vi "B7_65.vi"(4 "error in":T13, 7 "Command":T14) -> (0 "error out":T13, 3 "Response":T11)   [LabVIEW 2018]
uses:
  MOKO_LabViewLibrary/MokoLowLevel/MokoLowLovelControl/MLLC_Command.ctl
  MOKO_LabViewLibrary/MokoLowLevel/MokoLowLovelControl/MLLC_Error.ctl
  MOKO_LabViewLibrary/MokoLowLevel/MokoLowLovelControl/MLLC_Mode.ctl
  MOKO_LabViewLibrary/MokoLowLevel/MokoLowLovelControl/MLLC_Response.ctl
  MOKO_LabViewLibrary/MokoLowLevel/MokoLowLovelControl/MLLC_DriverName.ctl
  MOKO_LabViewLibrary/MokoLowLevel/MokoLowLovelControl/MLLC_ErrorCode.ctl
  MOKO_LabViewLibrary/MokoLowLevel/MokoLowLovelControl/MLLC_Request.ctl
  MOKO_LabViewLibrary/MokoLowLevel/MokoLowLovelControl/MLLC_ResponseInit.ctl
  MOKO_LabViewLibrary/MokoLowLevel/MokoLowLovelControl/MLLC_ConnectCluster.ctl
  MOKO_LabViewLibrary/MokoLowLevel/MokoLowLovelControl/MLLC_InterfaceType.ctl
  MOKO_LabViewLibrary/MokoLowLevel/MokoLowLovelControl/MLLC_OpenedSession.ctl
  MOKO_LabViewLibrary/MokoLowLevel/MokoLowLovelControl/MLLC_InterfaceSettings.ctl
  MOKO_LabViewLibrary/MokoLowLevel/MokoLowLovelControl/MLLC_InterfaceKind.ctl
  MOKO_LabViewLibrary/MokoLowLevel/MokoLowLovelControl/MLLC_Rs232Settings.ctl
panel:
  in  "Settings":T7={"Data"={"Connect"={"InterfaceType"=enum."VISA", "OpenedSession"="COM1", "InterfaceSettings"={"Interface"=enum."RS232", "EOS 4 read"=enum."LF (\\n)", "EOS 4 write"=enum."LF (\\n)", "TMO, ms"=10000, "Sett"=variant(cluster{"Baud Rate":u32, "Data Bits":u16, "Parity":u16, "Stop Bits":u16, "Flow Control":u16, "Eho":bool} {"Baud Rate"=75, "Data Bits"=0, "Parity"=0, "Stop Bits"=0, "Flow Control"=0, "Eho"=FALSE})}}, "Delay, ms"=100, "Function"=enum."VDC", "DIGITS"=enum."1"}, "Saved Data"=variant}
  in  "ResponseInit":T8
  in  "Request":T9
  in  "Error Code":T6=5424
  in  "Driver Name":T10="B7_65"
  in  "Mode":T12=enum."Check"
  # "B7-65"
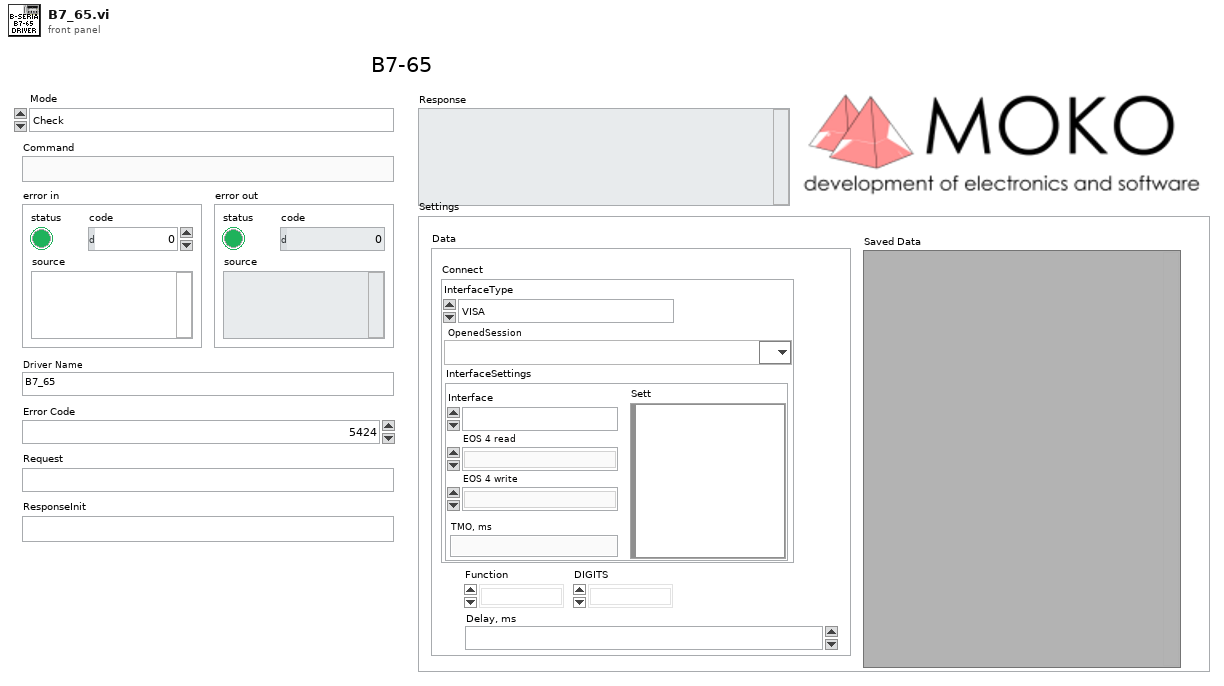
[diagram p1: front panel]
types:
  T1 = typedef "MLLC_ConnectCluster.ctl" = cluster{"InterfaceType":T2, "OpenedSession":T3, "InterfaceSettings":T4}
  T2 = typedef "MLLC_InterfaceType.ctl" = enum16{"VISA", "Prologix USB-GPIB"}
  T3 = typedef "MLLC_OpenedSession.ctl" = refnum<visa-resource-name>
  T4 = typedef "MLLC_InterfaceSettings.ctl" = cluster{"Interface":T5, "EOS 4 read":enum16{"Default (=EOS 4 write)", "CR (\\r)", "LF (\\n)", "None"}, "EOS 4 write":enum16{"CR+LF (\\r\\n)", "CR (\\r)", "LF (\\n)", "None"}, "TMO, ms":i32, "Sett":variant}
  T5 = typedef "MLLC_InterfaceKind.ctl" = enum16{"RS232", "GPIB", "USB", "Ethernet", "another"}
  T6 = typedef "MLLC_ErrorCode.ctl" = u32
  T7 = cluster{"Data":cluster{"Connect":T1, "Delay, ms":T6, "Function":enum16{"F", "T", "R4", "R", "IAC", "IDC", "VAC", "VDC"}, "DIGITS":enum16{"0", "1", "2"}}, "Saved Data":variant}
  T8 = typedef "MLLC_ResponseInit.ctl" = string
  T9 = typedef "MLLC_Request.ctl" = string
  T10 = typedef "MLLC_DriverName.ctl" = string
  T11 = typedef "MLLC_Response.ctl" = string
  T12 = typedef "MLLC_Mode.ctl" = enum16{"get", "set", "close", "Init", "Check"}
  T13 = typedef "MLLC_Error.ctl" = errorcluster
  T14 = typedef "MLLC_Command.ctl" = string
  T15 = cluster{"Connect":T1, "Delay, ms":T6, "Function":enum16{"F", "T", "R4", "R", "IAC", "IDC", "VAC", "VDC"}, "DIGITS":enum16{"0", "1", "2"}}
  T16 = enum16{"F", "T", "R4", "R", "IAC", "IDC", "VAC", "VDC"}
  T17 = typedef "MLLC_Rs232Settings.ctl" = cluster{"Baud Rate":u32, "Data Bits":u16, "Parity":u16, "Stop Bits":u16, "Flow Control":u16, "Eho":bool, "Address":dbl}
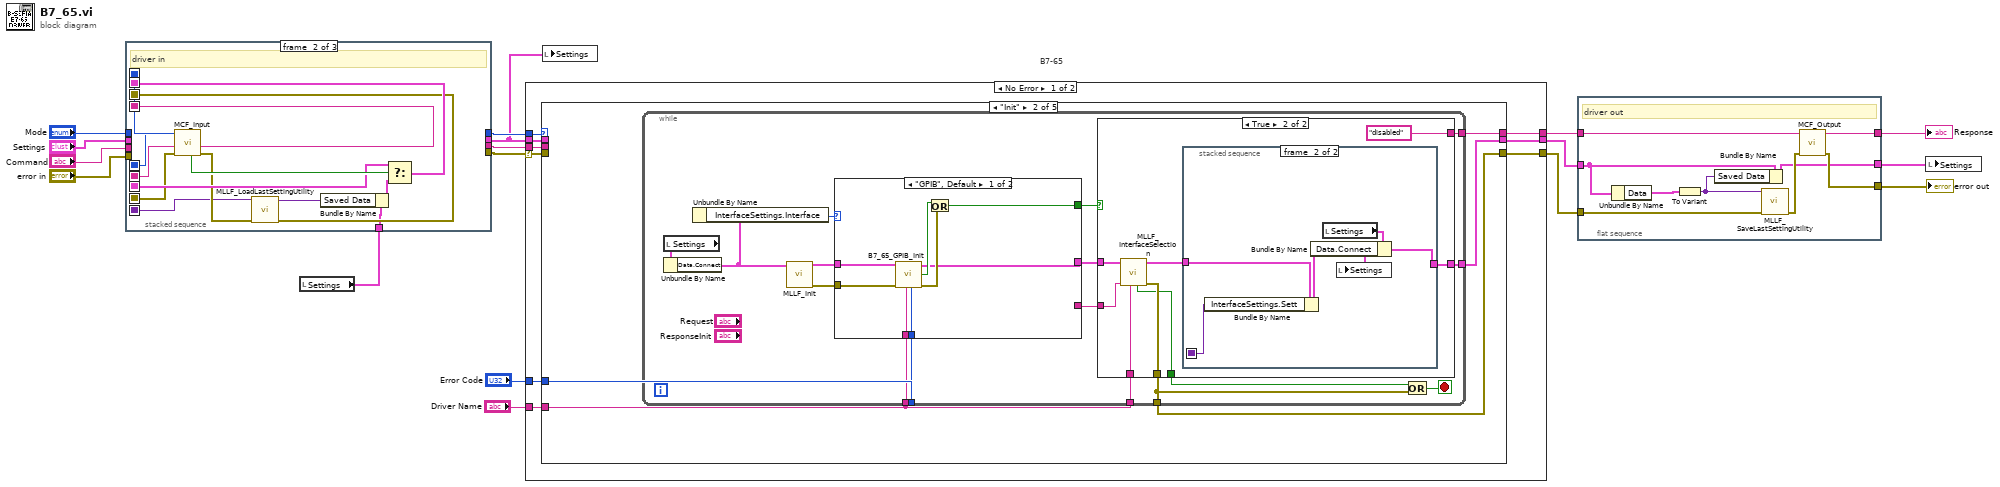
[diagram p0: block diagram]
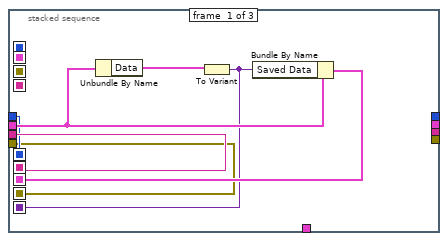
[diagram p2: hidden frame]
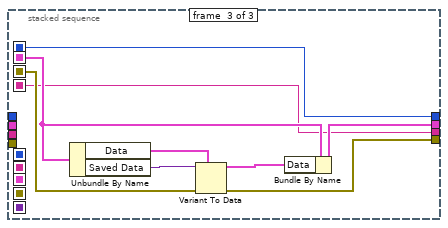
[diagram p3: hidden frame]
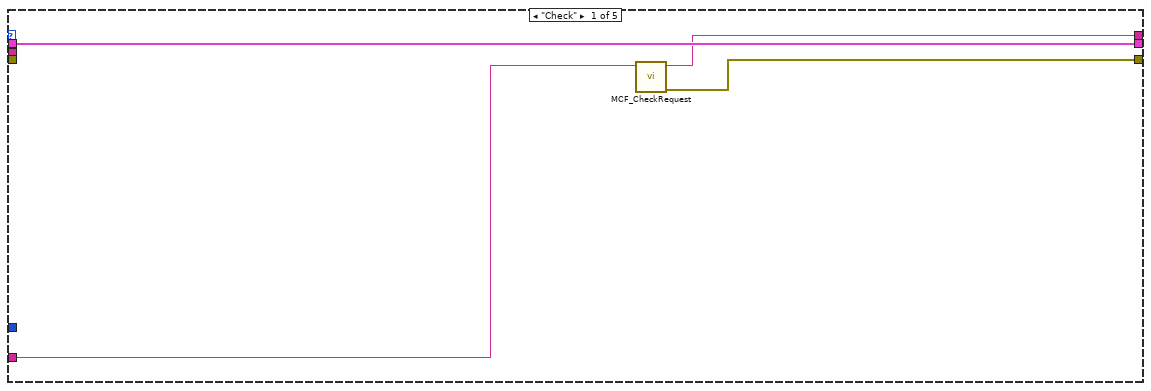
[diagram p4: hidden frame]
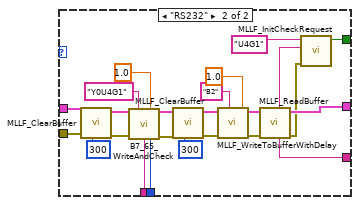
[diagram p5: hidden frame]
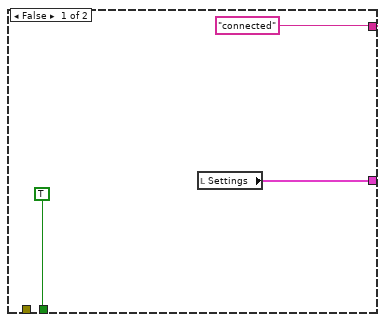
[diagram p6: hidden frame]
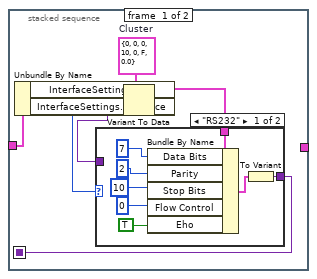
[diagram p7: hidden frame]
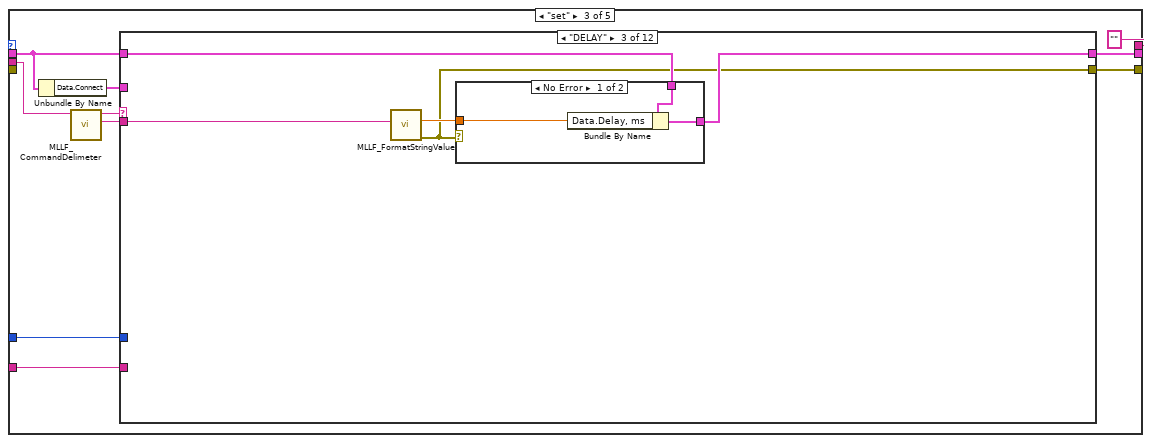
[diagram p9: hidden frame]
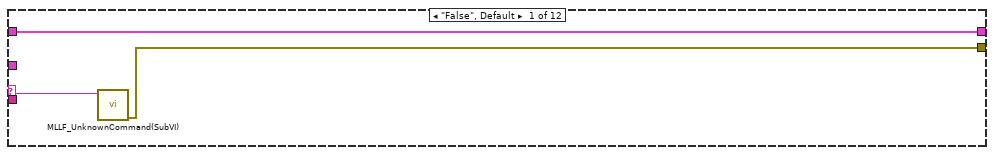
[diagram p10: hidden frame]
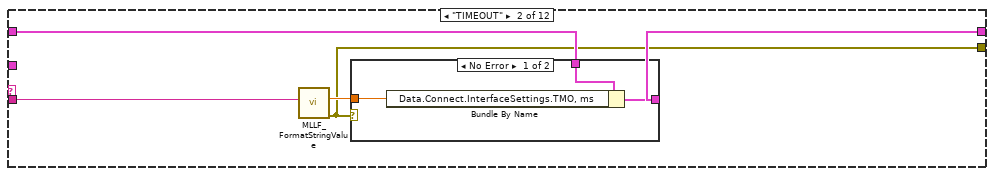
[diagram p11: hidden frame]
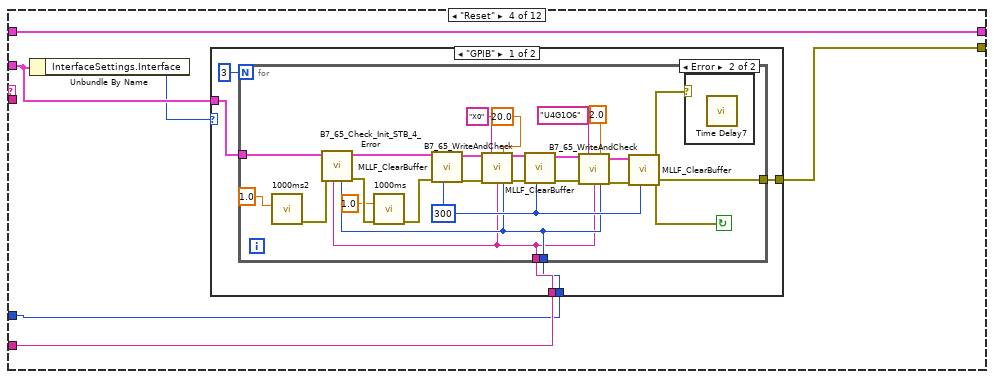
[diagram p14: hidden frame]
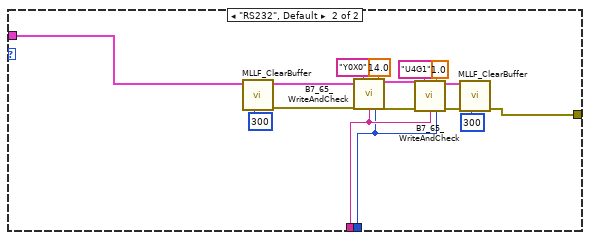
[diagram p16: hidden frame]
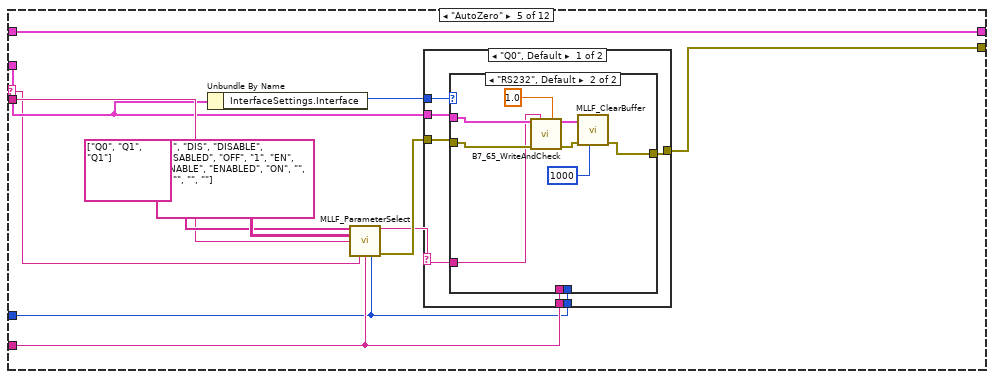
[diagram p17: hidden frame]
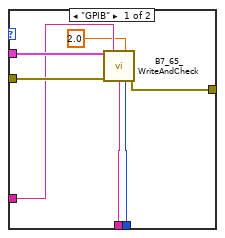
[diagram p18: hidden frame]
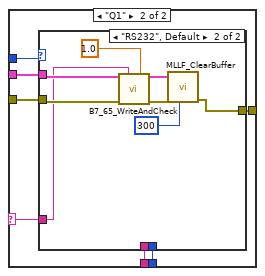
[diagram p19: hidden frame]
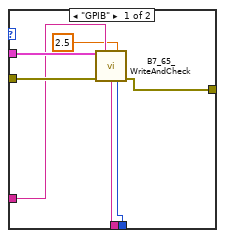
[diagram p20: hidden frame]
diagram:
  # "B7-65"
  n1 = local read "Settings"() -> (w11:T7)
  n2 = stacked-sequence {
    seq-local: [w20 _ _] -> [_ w36 _]
    seq-local: [w19 _ _] -> [_ w37 _]
    seq-local: [w22 _ _] -> [_ w32 _]
    seq-local: [w18 _ _] -> [_ w31 _]
    seq-local: [w21 _ _] -> [_ w27 _]
    seq-local: [_ w28 _] -> [_ _ w44]
    seq-local: [_ w38 _] -> [_ _ w41]
    seq-local: [_ w35 _] -> [_ _ w40]
    seq-local: [_ w34 _] -> [_ _ w45]
    tunnel: "Command" -> [w20 _ _]
    tunnel: "Mode" -> [w19 _ _]
    tunnel: "error in" -> [w18 _ _]
    tunnel: "Settings" -> [w23 _ _]
    tunnel: w11 -> [_ w26 _]
    tunnel: [_ _ w40] -> w8
    tunnel: [_ _ w43] -> w9
    tunnel: [_ _ w42] -> w7
    tunnel: [_ _ w41] -> w10
    frame #0 {
      n3 = Unbundle By Name(w23) -> ("Data"=w24:T15)
      n4 = To Variant(anything=w24) -> (Variant=w21:variant)
      n5 = Bundle By Name(cluster=w23, "Saved Data"=w21) -> (w22:T7)
    }
    frame #1 {
      # "driver in"
      n6 = call "MCF_Input.vi"("Error In"=w31, "Command in"=w36, "Mode in"=w37) -> ("Error Out"=w30:errorcluster, "Command out"=w35:string, "Mode out"=w38:T12, "Boolean"=w33:bool)  [unwired: 5 in]
      n7 = call "MLLF_LoadLastSettingUtility.vi"("Error In"=w30, "Save data in"=w27) -> ("Error Out"=w28:errorcluster, "Save data out"=w25:variant)  [unwired: 8 in]
      n8 = Bundle By Name(cluster=w26, "Saved Data"=w25) -> (w29:T7)
      n9 = Select(t=w32, s=w33, f=w29) -> (s? t:f=w34:T7)
    }
    frame #2 {
      n10 = Unbundle By Name(w45) -> ("Data"=w46:T15, "Saved Data"=w39:variant)
      n11 = Variant To Data(error in=w44, type=w46, Variant=w39) -> (data=w47:T15, error out=w42:errorcluster)
      n12 = Bundle By Name(cluster=w45, "Data"=w47) -> (w43:T7)
    }
  }
  n13 = case shown="No Error" w7 {
    selector: w7 -> [w52 w637]
    tunnel: [w54 w637] -> w4
    tunnel: w10 -> [w56 _]
    tunnel: [w55 _] -> w6
    tunnel: w8 -> [w53 _]
    tunnel: w9 -> [w49 w636]
    tunnel: "Error Code" -> [w51 _]
    tunnel: "Driver Name" -> [w50 _]
    tunnel: [w48 w636] -> w5
    frame No Error {
      n14 = case shown="\"Init\"" w56 {
        tunnel: [w59 w64 "" ("String") w417 "" ("String")] -> w55
        tunnel: [w58 w62 w144 w416 w634] -> w54
        tunnel: w53 -> [_ _ w153 w429 _]
        tunnel: w52 -> [_ _ _ _ _]
        tunnel: w51 -> [_ w65 w152 w426 _]
        tunnel: w50 -> [w57 w61 w149 w425 _]
        tunnel: w49 -> [w60 _ w151 w428 w633]
        tunnel: [w60 w63 w150 w427 w633] -> w48
        frame "Check" {
          n15 = call "MCF_CheckRequest.vi"("Driver Name"=w57) -> ("Error Out"=w58:errorcluster, "Output String"=w59:string)  [unwired: 9 in]
        }
        frame "Init" {
          n16 = while {
            tunnel: [w79] -> w62
            tunnel: w65 -> [w73]
            tunnel: w61 -> [w74]
            tunnel: [w71] -> w64
            tunnel: [w70] -> w63
            tunnel: w61 -> [w67]
            stop <- w78 stop-if-true
            n17 = local read "Settings"() -> (w81:T7)
            n18 = Unbundle By Name(w81) -> ("Data.Connect"=w68:T1)
            n19 = Unbundle By Name(w68) -> ("InterfaceSettings.Interface"=w72:T5)
            n20 = call "MLLF_Init.vi"("DriverConnect in"=w68) -> ("Error Out"=w75:errorcluster, "DriverConnect out"=w76:T1)  [unwired: 7 in]
            n21 = case shown="\"GPIB\", Default" w72 {
              tunnel: [w83 w112] -> w80
              tunnel: w76 -> [w88 w98]
              tunnel: w75 -> [w82 w97]
              tunnel: w74 -> [w87 w101]
              tunnel: w73 -> [w86 w100]
              tunnel: [w89 w93] -> w69
              tunnel: [_ w90] -> w66
              frame "GPIB", Default {
                n22 = call "B7_65_GPIB_Init.vi"("DriverConnect in"=w88, "error in"=w82, "Driver Name"=w87, "Error Code"=w86) -> ("DriverConnect out"=w83:T1, "Not Found response"=w84:bool, "error out"=w85:T13)  [unwired: 9 in]
                n23 = Or(x=w84, y=w85) -> (x .or. y?=w89:bool)
              }
              frame "RS232" {
                n24 = call "MLLF_ClearBuffer.vi"("Timeout(default = 300 ms)"=u32 300 ("Timeout"), "Error In"=w97, "DriverConnect in"=w98) -> ("Error Out"=w95:errorcluster, "DriverConnect out"=w96:T1)  [unwired: 5 in, 1 out]
                n25 = call "B7_65_WriteAndCheck.vi"("DriverConnect in"=w96, "Str2Write"="Y0U4G1" ("Request"), "Command Time (s)"=1.0, "error in"=w95, "Driver Name"=w101, "Error Code"=w100) -> ("DriverConnect out"=w104:T1, "error out"=w103:T13)  [unwired: 8 in]
                n26 = call "MLLF_ClearBuffer.vi"("Timeout(default = 300 ms)"=u32 300 ("Timeout"), "Error In"=w103, "DriverConnect in"=w104) -> ("Error Out"=w108:errorcluster, "DriverConnect out"=w109:T1)  [unwired: 5 in, 1 out]
                n27 = call "MLLF_WriteToBufferWithDelay.vi"("Delay Time ( 0,05 s)"=1.0 ("Command Time (s)"), "Command"="B2" ("Request"), "Error In"=w108, "DriverConnect in"=w109) -> ("Error Out"=w105:errorcluster, "DriverConnect out"=w106:T1)  [unwired: 6 in]
                n28 = call "MLLF_ReadBuffer.vi"("Error In"=w105, "DriverConnect in"=w106) -> ("Error Out"=w91:errorcluster, "DriverConnect out"=w112:T1, "String"=w90:string)  [unwired: 6 in]
                n29 = call "MLLF_InitCheckRequest.vi"("error in (no error)"=w91, "Answer"=w90, "Response Init"="U4G1" ("Response")) -> ("Design"=w93:bool)  [unwired: 5 in, 3 out]
              }
            }
            n30 = case shown="True" w69 {
              tunnel: w80 -> [_ w123]
              tunnel: [_ w121] -> w79
              tunnel: [TRUE w120] -> w77
              tunnel: [w113 w119] -> w70
              tunnel: ["connected" "disabled"] -> w71
              tunnel: w67 -> [_ w117]
              tunnel: w66 -> [_ w116]
              frame False {
                n31 = local read "Settings"() -> (w113:T7)
              }
              frame True {
                n32 = call "MLLF_InterfaceSelection.vi"("Driver Name"=w117, "Answer:"=w116, "DriverConnect in"=w123) -> ("error out"=w121:T13, "DriverConnect out"=w122:T1, "stop init?"=w120:bool)  [unwired: 4 in, 2 out]
                n33 = stacked-sequence {
                  seq-local: [w127 _] -> [_ w142]
                  tunnel: w122 -> [w124 w140]
                  tunnel: [_ w141] -> w119
                  frame #0 {
                    w129 = T17 {"Baud Rate"=0, "Data Bits"=0, "Parity"=0, "Stop Bits"=10, "Flow Control"=0, "Eho"=FALSE, "Address"=0.0}  # Cluster
                    n34 = Unbundle By Name(w124) -> ("InterfaceSettings.Sett"=w126:variant, "InterfaceSettings.Interface"=w125:T5)
                    n35 = Variant To Data(type=w129, Variant=w126) -> (data=w128:T17)  [unwired: 1 in, 1 out]
                    n36 = case shown="\"RS232\"" w125 {
                      tunnel: w128 -> [w136 _]
                      tunnel: [w137 w138] -> w127
                      tunnel: w126 -> [_ w138]
                      frame "RS232" {
                        n37 = Bundle By Name(cluster=w136, "Data Bits"=u16 7 ("Serial Settings:Data Bits"), "Parity"=u16 2 ("Flow Control"), "Stop Bits"=u16 10 ("Flow Control"), "Flow Control"=u16 0, "Eho"=TRUE) -> (w135:T17)
                        n38 = To Variant(anything=w135) -> (Variant=w137:variant)
                      }
                      frame "GPIB", Default {
                      }
                    }
                  }
                  frame #1 {
                    n39 = Bundle By Name(cluster=w140, "InterfaceSettings.Sett"=w142) -> (w139:T1)
                    n40 = local read "Settings"() -> (w143:T7)
                    n41 = Bundle By Name(cluster=w143, "Data.Connect"=w139) -> (w141:T7)
                    n42 = local write "Settings"(w141) -> ()
                  }
                }
              }
            }
            n43 = Or(x=w77, y=w79) -> (x .or. y?=w78:bool)
          }
        }
        frame "set" {
          n44 = Unbundle By Name(w151) -> ("Data.Connect"=w147:T1)
          n45 = call "MLLF_CommandDelimeter.vi"("command with param"=w153) -> ("param 1"=w145:string, "command"=w146:string)  [unwired: 6 in, 3 out]
          n46 = case shown="\"DELAY\"" w146 {
            selector: w146 -> [w155 _ _ _ w225 w281 _ w297 _ _ w378 w390]
            tunnel: w145 -> [_ w159 w168 _ w233 w291 _ w319 w333 _ w386 w404]
            tunnel: [w154 w157 w166 w180 w230 w288 _ w306 w334 _ w380 w393] -> w144
            tunnel: w152 -> [_ _ _ w177 w228 w286 _ w311 w339 _ w385 w400]
            tunnel: w151 -> [w156 w160 w169 w179 w236 w295 w296 w316 w351 w377 w389 w392]
            tunnel: [w156 w161 w170 w179 w236 w295 w296 w317 w351 w377 w389 w391] -> w150
            tunnel: w147 -> [_ _ _ w176 w226 w292 _ w298 w338 _ w383 w403]
            tunnel: w149 -> [_ _ _ w178 w229 w287 _ w312 w340 _ w384 w401]
            frame "False", Default {
              n47 = call "MLLF_UnknownCommand(SubVI).vi"("Unknown command"=w155) -> ("error out"=w154:errorcluster)  [unwired: 10 in]
            }
            frame "TIMEOUT" {
              n48 = call "MLLF_FormatStringValue.vi"("String Value"=w159) -> ("error out"=w157:T13, "number"=w158:dbl)  [unwired: 8 in, 1 out]
              n49 = case shown="No Error" w157 {
                tunnel: [w164 w165] -> w161
                tunnel: w160 -> [w163 w165]
                tunnel: w158 -> [w162 _]
                frame No Error {
                  n50 = Bundle By Name(cluster=w163, "Data.Connect.InterfaceSettings.TMO, ms"=w162) -> (w164:T7)
                }
                frame Error {
                }
              }
            }
            frame "DELAY" {
              n51 = call "MLLF_FormatStringValue.vi"("String Value"=w168) -> ("error out"=w166:T13, "number"=w167:dbl)  [unwired: 8 in, 1 out]
              n52 = case shown="No Error" w166 {
                tunnel: [w173 w174] -> w170
                tunnel: w169 -> [w172 w174]
                tunnel: w167 -> [w171 _]
                frame No Error {
                  n53 = Bundle By Name(cluster=w172, "Data.Delay, ms"=w171) -> (w173:T7)
                }
                frame Error {
                }
              }
            }
            frame "Reset" {
              n54 = Unbundle By Name(w176) -> ("InterfaceSettings.Interface"=w175:T5)
              n55 = case shown="\"GPIB\"" w175 {
                tunnel: w178 -> [w183 w218]
                tunnel: w177 -> [w182 w217]
                tunnel: [w185 w224] -> w180
                tunnel: w176 -> [w184 w209]
                frame "GPIB" {
                  n56 = for {
                    N: 3 -> [_]
                    tunnel: [w194] -> w185
                    tunnel: w184 -> [w193]
                    tunnel: w183 -> [w191]
                    tunnel: w182 -> [w192]
                    stop <- w194 continue-if-true
                    w196 = u32 300 ("Timeout")
                    n57 = call "1000ms2"("Delay Time (s)"=1.0 ("Command Time (s)")) -> ("error out"=w188:errorcluster)  [unwired: 10 in]
                    n58 = call "B7_65_Check_Init_STB_4_Error.vi"("Error Code"=w192, "Driver Name"=w191, "error in"=w188, "DriverConnect in"=w193) -> ("error out"=w190:T13, "DriverConnect out"=w195:T1)  [unwired: 6 in]
                    n59 = call "1000ms"("error in (no error)"=w190, "Delay Time (s)"=1.0 ("Command Time (s)")) -> ("error out"=w189:errorcluster)  [unwired: 9 in]
                    n60 = call "MLLF_ClearBuffer.vi"("Timeout(default = 300 ms)"=w196, "Error In"=w189, "DriverConnect in"=w195) -> ("Error Out"=w199:errorcluster, "DriverConnect out"=w200:T1)  [unwired: 5 in, 1 out]
                    n61 = call "B7_65_WriteAndCheck.vi"("DriverConnect in"=w200, "Str2Write"="X0", "Command Time (s)"=20.0, "error in"=w199, "Driver Name"=w191, "Error Code"=w192) -> ("DriverConnect out"=w206:T1, "error out"=w205:T13)  [unwired: 8 in]
                    n62 = call "MLLF_ClearBuffer.vi"("Timeout(default = 300 ms)"=w196, "Error In"=w205, "DriverConnect in"=w206) -> ("Error Out"=w203:errorcluster, "DriverConnect out"=w204:T1)  [unwired: 5 in, 1 out]
                    n63 = call "B7_65_WriteAndCheck.vi"("DriverConnect in"=w204, "Str2Write"="U4G1O6" ("Request"), "Command Time (s)"=2.0, "error in"=w203, "Driver Name"=w191, "Error Code"=w192) -> ("DriverConnect out"=w198:T1, "error out"=w197:T13)  [unwired: 8 in]
                    n64 = call "MLLF_ClearBuffer.vi"("Timeout(default = 300 ms)"=w196, "Error In"=w197, "DriverConnect in"=w198) -> ("Error Out"=w194:errorcluster)  [unwired: 5 in, 2 out]
                    n65 = case shown="Error" w194 {
                      frame No Error {
                      }
                      frame Error {
                        n66 = call "Time Delay7"() -> ()  [unwired: 11 in, 1 out]
                      }
                    }
                  }
                }
                frame "RS232", Default {
                  n67 = call "MLLF_ClearBuffer.vi"("Timeout(default = 300 ms)"=u32 300 ("Timeout"), "DriverConnect in"=w209) -> ("Error Out"=w210:errorcluster, "DriverConnect out"=w211:T1)  [unwired: 6 in, 1 out]
                  n68 = call "B7_65_WriteAndCheck.vi"("DriverConnect in"=w211, "Str2Write"="Y0X0" ("Request"), "Command Time (s)"=14.0, "error in"=w210, "Driver Name"=w218, "Error Code"=w217) -> ("DriverConnect out"=w222:T1, "error out"=w221:T13)  [unwired: 8 in]
                  n69 = call "B7_65_WriteAndCheck.vi"("DriverConnect in"=w222, "Str2Write"="U4G1" ("Request"), "Command Time (s)"=1.0, "error in"=w221, "Driver Name"=w218, "Error Code"=w217) -> ("DriverConnect out"=w220:T1, "error out"=w219:T13)  [unwired: 8 in]
                  n70 = call "MLLF_ClearBuffer.vi"("Timeout(default = 300 ms)"=u32 300 ("Timeout"), "Error In"=w219, "DriverConnect in"=w220) -> ("Error Out"=w224:errorcluster)  [unwired: 5 in, 2 out]
                }
              }
            }
            frame "AutoZero" {
              n71 = Unbundle By Name(w226) -> ("InterfaceSettings.Interface"=w227:T5)
              n72 = call "MLLF_ParameterSelect.vi"("Command to equipment"=string[] ["Q0", "Q1", "Q1"] ("Names"), "Names"=string[][] [["0", "DIS", "DISABLE", "DISABLED", "OFF"], ["1", "EN", "ENABLE", "ENABLED", "ON"], ["", "", "", "", ""]], "Input"=w233, "Command"=w225, "Driver Name"=w229, "Error Code"=w228) -> ("Choice"=w231:string, "Error Out"=w232:errorcluster)  [unwired: 8 in]
              n73 = case shown="\"Q0\", Default" w231 {
                selector: w231 -> [w241 w265]
                tunnel: w226 -> [w243 w260]
                tunnel: [w240 w264] -> w230
                tunnel: w232 -> [w242 w261]
                tunnel: w229 -> [w239 w262]
                tunnel: w228 -> [w238 w263]
                tunnel: w227 -> [w237 w259]
                frame "Q0", Default {
                  n74 = case shown="\"RS232\", Default" w237 {
                    tunnel: w241 -> [w248 w252]
                    tunnel: [w247 w258] -> w240
                    tunnel: w242 -> [w249 w255]
                    tunnel: w243 -> [w250 w256]
                    tunnel: w239 -> [w245 _]
                    tunnel: w238 -> [w244 _]
                    frame "GPIB" {
                      n75 = call "B7_65_WriteAndCheck.vi"("DriverConnect in"=w250, "Str2Write"=w248, "Command Time (s)"=2.0, "error in"=w249, "Driver Name"=w245, "Error Code"=w244) -> ("error out"=w247:T13)  [unwired: 8 in, 1 out]
                    }
                    frame "RS232", Default {
                      n76 = call "B7_65_WriteAndCheck.vi"("DriverConnect in"=w256, "Str2Write"=w252, "Command Time (s)"=1.0, "error in"=w255) -> ("DriverConnect out"=w254:T1, "error out"=w253:T13)  [unwired: 10 in]
                      n77 = call "MLLF_ClearBuffer.vi"("Timeout(default = 300 ms)"=u32 1000 ("Timeout"), "Error In"=w253, "DriverConnect in"=w254) -> ("Error Out"=w258:errorcluster)  [unwired: 5 in, 2 out]
                    }
                  }
                }
                frame "Q1" {
                  n78 = case shown="\"RS232\", Default" w259 {
                    tunnel: w265 -> [w270 w274]
                    tunnel: [w267 w280] -> w264
                    tunnel: w263 -> [w268 _]
                    tunnel: w262 -> [w269 _]
                    tunnel: w261 -> [w271 w277]
                    tunnel: w260 -> [w272 w278]
                    frame "GPIB" {
                      n79 = call "B7_65_WriteAndCheck.vi"("DriverConnect in"=w272, "Str2Write"=w270, "Command Time (s)"=2.5, "error in"=w271, "Driver Name"=w269, "Error Code"=w268) -> ("error out"=w267:T13)  [unwired: 8 in, 1 out]
                    }
                    frame "RS232", Default {
                      n80 = call "B7_65_WriteAndCheck.vi"("DriverConnect in"=w278, "Str2Write"=w274, "Command Time (s)"=1.0, "error in"=w277) -> ("DriverConnect out"=w276:T1, "error out"=w275:T13)  [unwired: 10 in]
                      n81 = call "MLLF_ClearBuffer.vi"("Timeout(default = 300 ms)"=u32 300 ("Timeout"), "Error In"=w275, "DriverConnect in"=w276) -> ("Error Out"=w280:errorcluster)  [unwired: 5 in, 2 out]
                    }
                  }
                }
              }
            }
            frame "Calibr", "Calibration" {
              n82 = call "MLLF_ParameterSelect.vi"("Command to equipment"=string[] ["K0"] ("Names"), "Names"=string[][] [["1", "EN", "ENABLE", "ENABLEÂ", "ON"], ["", "", "", "", ""], ["", "", "", "", ""]], "Input"=w291, "Command"=w281, "Driver Name"=w287, "Error Code"=w286) -> ("Choice"=w289:string, "Error Out"=w290:errorcluster)  [unwired: 8 in]
              n83 = call "B7_65_WriteAndCheck.vi"("DriverConnect in"=w292, "Str2Write"=w289, "Command Time (s)"=14.0 ("Delay Time (s)"), "error in"=w290, "Driver Name"=w287, "Error Code"=w286) -> ("DriverConnect out"=w283:T1, "error out"=w282:T13)  [unwired: 8 in]
              n84 = call "MLLF_ClearBuffer.vi"("Timeout(default = 300 ms)"=u32 300 ("Timeout"), "Error In"=w282, "DriverConnect in"=w283) -> ("Error Out"=w288:errorcluster)  [unwired: 5 in, 2 out]
            }
            frame "--------------------Main----------------------" {
            }
            frame "Func", "Function" {
              n85 = call "MLLF_ClearBuffer.vi"("Timeout(default = 300 ms)"=u32 300 ("Timeout"), "DriverConnect in"=w298) -> ("Error Out"=w302:errorcluster, "DriverConnect out"=w301:T1)  [unwired: 6 in, 1 out]
              n86 = call "B7_65_WriteAndCheck.vi"("DriverConnect in"=w301, "Str2Write"="Q0H1" ("Request"), "Command Time (s)"=2.0, "error in"=w302) -> ("DriverConnect out"=w300:T1, "error out"=w299:T13)  [unwired: 10 in]
              n87 = call "MLLF_ParameterSelect.vi"("Command to equipment"=string[] ["U4", "V4", "I1", "J1", "R1", "Z1", "F0", "T0"] ("Names"), "Names"=string[][] [["VDC", "", ""], ["VAC", "", ""], ["IDC", "", ""], ["IAC", "", ""], ["R", "R2", "R2WIRE"], ["R4", "R4WIRE", ""], ["F", "FREQ", ""], ["T", "P", "PERIOD"]], "Input"=w319, "Error In"=w299, "Command"=w297, "Driver Name"=w312, "Error Code"=w311) -> ("Choice"=w314:string, "Error Out"=w310:errorcluster)  [unwired: 7 in]
              n88 = case shown="\"T0\"" w314 {
                tunnel: [_ T16."VDC" ("Function") T16."VAC" ("Function") T16."IDC" ("Function") T16."IAC" ("Function") T16."R" ("Function") T16."R4" ("Function") T16."F" ("Function") T16."T" ("Function")] -> w315
                frame "False", Default {
                }
                frame "U4" {
                }
                frame "V4" {
                }
                frame "I1" {
                }
                frame "J1" {
                }
                frame "R1" {
                }
                frame "Z1" {
                }
                frame "F0" {
                }
                frame "T0" {
                }
              }
              n89 = call "B7_65_WriteAndCheck.vi"("DriverConnect in"=w300, "Str2Write"=w314, "Command Time (s)"=2.0 ("Delay Time (s)"), "error in"=w310, "Driver Name"=w312, "Error Code"=w311) -> ("DriverConnect out"=w308:T1, "error out"=w307:T13)  [unwired: 8 in]
              n90 = call "MLLF_ClearBuffer.vi"("Timeout(default = 300 ms)"=u32 300 ("Timeout"), "Error In"=w307, "DriverConnect in"=w308) -> ("Error Out"=w306:errorcluster)  [unwired: 5 in, 2 out]
              n91 = case shown="No Error" w306 {
                tunnel: [w331 w332] -> w317
                tunnel: w316 -> [w330 w332]
                tunnel: w315 -> [w329 _]
                frame No Error {
                  n92 = Bundle By Name(cluster=w330, "Data.Function"=w329) -> (w331:T7)
                }
                frame Error {
                }
              }
            }
            frame "RANGE" {
              # "Q0 - autozero off"
              n93 = Unbundle By Name(w351) -> ("Data.Function"=w352:T16)
              n94 = Index Array(array=string[] ["F", "T", "Z", "R", "J", "I", "V", "U"] ("Names"), index=w352) -> (element=w336:string)
              n95 = case shown="\"1\", Default" w333 {
                selector: w333 -> [w353 _]
                tunnel: [w355 _] -> w344
                tunnel: [w357 "1A1" ("String")] -> w350
                tunnel: w336 -> [w358 _]
                tunnel: [w354 1.0 ("Delay Time (s)")] -> w337
                frame "1", Default {
                  n96 = call "MLLF_FormatStringValue.vi"("String Value"=w353) -> ("error out"=w355:T13, "number"=w356:dbl)  [unwired: 8 in, 1 out]
                  n97 = case shown="\"R\", \"Z\"" w358 {
                    tunnel: [w364 w372 "1" ("Request")] -> w357
                    tunnel: w356 -> [w361 w370 _]
                    tunnel: [w359 2.0 ("Delay Time (s)") 2.0 ("Delay Time (s)")] -> w354
                    frame "R", "Z" {
                      n98 = Less?(x=w361, y=2000000.0) -> (x < y?=w360:bool)
                      n99 = call "B7_65_StandartRangeSelect (SubVI).vi"("Control Point"=w361, "RangeDigit"=dbl[] [200.0, 2000.0, 20000.0, 200000.0, 2000000.0, 20000000.0, 2000000000.0, 2000000000.0], "RangeCommand"=string[] ["0", "1", "2", "3", "4", "5", "6", ""]) -> ("R/O"=w364:string)  [unwired: 1 in]
                      n100 = case shown="True" w360 {
                        tunnel: [2.0 ("Delay Time (s)") 10.0 ("Delay Time (s)")] -> w359
                        frame True {
                        }
                        frame False {
                        }
                      }
                    }
                    frame "U", "V", Default {
                      n101 = call "B7_65_StandartRangeSelect (SubVI).vi"("Control Point"=w370, "RangeDigit"=dbl[] [0.2, 2.0, 20.0, 200.0, 2000.0], "RangeCommand"=string[] ["0", "1", "2", "3", "4"]) -> ("R/O"=w372:string)  [unwired: 1 in]
                    }
                    frame "I", "J" {
                    }
                  }
                }
                frame "auto" {
                }
              }
              n102 = Concatenate Strings(w336, w350) -> (w349:string)
              n103 = call "MLLF_ClearBuffer.vi"("Timeout(default = 300 ms)"=u32 300 ("Timeout"), "Error In"=w344, "DriverConnect in"=w338) -> ("Error Out"=w343:errorcluster, "DriverConnect out"=w341:T1)  [unwired: 5 in, 1 out]
              n104 = call "B7_65_WriteAndCheck.vi"("DriverConnect in"=w341, "Str2Write"="Q0" ("Request"), "Command Time (s)"=1.0, "error in"=w343, "Driver Name"=w340, "Error Code"=w339) -> ("DriverConnect out"=w345:T1, "error out"=w342:T13)  [unwired: 8 in]
              n105 = call "B7_65_WriteAndCheck.vi"("DriverConnect in"=w345, "Str2Write"=w349, "Command Time (s)"=w337, "error in"=w342, "Driver Name"=w340, "Error Code"=w339) -> ("error out"=w334:T13)  [unwired: 8 in, 1 out]
            }
            frame "-------------Supplemental------------" {
            }
            frame "ACQ", "ACQUISITION" {
              n106 = call "MLLF_ParameterSelect.vi"("Command to equipment"=string[] ["T0", "T1"] ("Names"), "Names"=string[][] [["CONT", "CONTINUOUS", ""], ["ONCE", "ONETIME", "1"]], "Input"=w386, "Command"=w378, "Driver Name"=w384, "Error Code"=w385) -> ("Choice"=w382:string, "Error Out"=w381:errorcluster)  [unwired: 8 in]
              n107 = call "B7_65_WriteAndCheck.vi"("DriverConnect in"=w383, "Str2Write"=w382, "Command Time (s)"=1.0 ("Delay Time (s)"), "error in"=w381, "Driver Name"=w384, "Error Code"=w385) -> ("error out"=w380:T13)  [unwired: 8 in, 1 out]
            }
            frame "DIGITS", "DISP", "DISPLAY", "INTEGRATIONTIME", "INTTIME" {
              n108 = call "MLLF_ParameterSelect.vi"("Command to equipment"=string[] ["H2", "H1", "H0"] ("Names"), "Names"=string[][] [["5.5", "5,5", "6"], ["4.5", "4,5", "5"], ["3.5", "3,5", "4"]], "Input"=w404, "Command"=w390, "Driver Name"=w401, "Error Code"=w400) -> ("Choice"=w394:string, "Error Out"=w402:errorcluster)  [unwired: 8 in]
              n109 = case shown="\"H2\"" w394 {
                tunnel: [_ enum16{"0", "1", "2"}."0" ("Function") enum16{"0", "1", "2"}."1" ("Function") enum16{"0", "1", "2"}."2" ("Function")] -> w395
                frame "False", Default {
                }
                frame "H0" {
                }
                frame "H1" {
                }
                frame "H2" {
                }
              }
              n110 = call "B7_65_WriteAndCheck.vi"("DriverConnect in"=w403, "Str2Write"=w394, "Command Time (s)"=2.0 ("Delay Time (s)"), "error in"=w402, "Driver Name"=w401, "Error Code"=w400) -> ("DriverConnect out"=w397:T1, "error out"=w396:T13)  [unwired: 8 in]
              n111 = call "MLLF_ClearBuffer.vi"("Timeout(default = 300 ms)"=u32 300 ("Timeout"), "Error In"=w396, "DriverConnect in"=w397) -> ("Error Out"=w393:errorcluster)  [unwired: 5 in, 2 out]
              n112 = case shown="No Error" w393 {
                tunnel: [w412 w413] -> w391
                tunnel: w392 -> [w411 w413]
                tunnel: w395 -> [w410 _]
                frame No Error {
                  n113 = Bundle By Name(cluster=w411, "Data.DIGITS"=w410) -> (w412:T7)
                }
                frame Error {
                }
              }
            }
          }
        }
        frame "get" {
          n114 = Unbundle By Name(w428) -> ("Data.Connect"=w423:T1, "Data.Function"=w421:T16)
          n115 = call "MLLF_CommandDelimeter.vi"("command with param"=w429) -> ("param 1"=w414:string, "command"=w415:string)  [unwired: 6 in, 3 out]
          n116 = call "B7_65_Choice_function_and_digits.vi"("Settings"=w428) -> ("Digits"=w419:string, "Function"=w420:string)  [unwired: 9 in]
          n117 = case shown="\"False\", Default" w415 {
            selector: w415 -> [w431 _ _]
            tunnel: w414 -> [_ _ w438]
            tunnel: [w430 _ w459] -> w418
            tunnel: w426 -> [_ _ w443]
            tunnel: [w434 w437 w460] -> w427
            tunnel: w428 -> [w434 w437 w460]
            tunnel: [w432 w435 w446] -> w424
            tunnel: w423 -> [_ _ w440]
            tunnel: w425 -> [_ _ w444]
            tunnel: w421 -> [_ _ _]
            tunnel: w420 -> [_ _ w445]
            tunnel: w419 -> [_ _ w441]
            frame "False", Default {
              n118 = call "MLLF_UnknownCommand(SubVI).vi"("Unknown command"=w431) -> ("error out"=w430:errorcluster)  [unwired: 10 in]
              n119 = Build Array(0 ("TimeOut")) -> (w432:i32[])
            }
            frame "TIMEOUT" {
              n120 = Unbundle By Name(w437) -> ("Data.Connect.InterfaceSettings.TMO, ms"=w436:i32)
              n121 = Build Array(w436) -> (w435:i32[])
            }
            frame "FETCH", "READ" {
              n122 = Unbundle By Name(w440) -> ("InterfaceSettings.Interface"=w439:T5)
              n123 = call "MLLF_ClearBuffer.vi"("Timeout(default = 300 ms)"=u32 300 ("Timeout"), "DriverConnect in"=w440) -> ("Error Out"=w448:errorcluster, "DriverConnect out"=w447:T1)  [unwired: 6 in, 1 out]
              n124 = Decimal String To Number(string=w438) -> (number=w458:i32)  [unwired: 2 in, 1 out]
              n125 = In Range and Coerce(upper limit=100, x=w458, lower limit=1) -> (coerced(x)=w442:i32)  [unwired: 1 out]
              n126 = case shown="\"GPIB\", Default" w439 {
                tunnel: [w468 w531] -> w450
                tunnel: w447 -> [w470 w535]
                tunnel: w448 -> [w469 w534]
                tunnel: [w463 w532] -> w451
                tunnel: [w467 w530] -> w449
                tunnel: w442 -> [w464 w533]
                tunnel: w445 -> [w471 w529]
                tunnel: w443 -> [w466 w525]
                tunnel: w444 -> [w465 w526]
                tunnel: w444 -> [w462 w528]
                tunnel: w443 -> [w461 w527]
                tunnel: w441 -> [_ w524]
                frame "RS232" {
                  n127 = case shown="\"F\", \"T\"" w471 {
                    tunnel: w470 -> [w479 w508]
                    tunnel: w469 -> [w478 w507]
                    tunnel: [w485 w506] -> w468
                    tunnel: [w484 w505] -> w467
                    tunnel: w466 -> [w483 w504]
                    tunnel: w465 -> [w482 w502]
                    tunnel: w464 -> [w481 w503]
                    tunnel: [w480 w501] -> w463
                    tunnel: w462 -> [w473 _]
                    tunnel: w461 -> [w472 _]
                    frame "I", "J", "R", "U", "V", "Z", Default {
                      n128 = call "B7_65_WriteAndCheck.vi"("DriverConnect in"=w479, "Str2Write"="B1" ("String"), "Command Time (s)"=0.5, "error in"=w478, "Driver Name"=w473, "Error Code"=w472) -> ("DriverConnect out"=w477:T1, "error out"=w476:T13)  [unwired: 8 in]
                      n129 = for {
                        N: w481 -> [_]
                        tunnel: [w499] -> w480 mode=indexing
                        tunnel: [w498] -> w487
                        tunnel: [w496] -> w486
                        tunnel: w477 -> [w492]
                        tunnel: w476 -> [w493]
                        stop <- w498 stop-if-true
                        n130 = call "MLLF_WriteToBufferWithDelay.vi"("Delay Time ( 0,05 s)"=0.1 ("Command Time (s)"), "Command"="X1" ("String"), "Error In"=w493, "DriverConnect in"=w492) -> ("Error Out"=w494:errorcluster, "DriverConnect out"=w495:T1)  [unwired: 6 in]
                        n131 = call "MLLF_ReadBuffer.vi"("Error In"=w494, "DriverConnect in"=w495) -> ("Error Out"=w498:errorcluster, "DriverConnect out"=w496:T1, "String"=w497:string)  [unwired: 6 in]
                        n132 = Fract/Exp String To Number(use system decimal point (T)=FALSE, string=w497) -> (number=w499:dbl)  [unwired: 2 in, 1 out]
                      }
                      n133 = call "B7_65_WriteAndCheck.vi"("DriverConnect in"=w486, "Str2Write"="G1B0" ("String"), "Command Time (s)"=0.5, "error in"=w487, "Driver Name"=w482, "Error Code"=w483) -> ("DriverConnect out"=w485:T1, "error out"=w484:T13)  [unwired: 8 in]
                    }
                    frame "F", "T" {
                      n134 = call "MLLF_WriteToBufferWithDelay.vi"("Delay Time ( 0,05 s)"=0.5 ("Command Time (s)"), "Command"="G0B1" ("String"), "Error In"=w507, "DriverConnect in"=w508) -> ("Error Out"=w514:errorcluster, "DriverConnect out"=w515:T1)  [unwired: 6 in]
                      n135 = for {
                        N: w503 -> [_]
                        tunnel: [w522] -> w501 mode=indexing
                        tunnel: [w521] -> w509
                        tunnel: [w519] -> w510
                        tunnel: w515 -> [w518]
                        tunnel: w514 -> [w517]
                        stop <- w521 stop-if-true
                        n136 = call "MLLF_ReadBuffer.vi"("Error In"=w517, "DriverConnect in"=w518) -> ("Error Out"=w521:errorcluster, "DriverConnect out"=w519:T1, "String"=w520:string)  [unwired: 6 in]
                        n137 = Fract/Exp String To Number(use system decimal point (T)=FALSE, string=w520) -> (number=w522:dbl)  [unwired: 2 in, 1 out]
                      }
                      n138 = call "B7_65_WriteAndCheck.vi"("DriverConnect in"=w510, "Str2Write"="G1B0" ("String"), "Command Time (s)"=0.5, "error in"=w509, "Driver Name"=w502, "Error Code"=w504) -> ("DriverConnect out"=w506:T1, "error out"=w505:T13)  [unwired: 8 in]
                    }
                  }
                }
                frame "GPIB", Default {
                  n139 = case shown="\"I\", \"J\", \"U\", \"V\", Default" w529 {
                    tunnel: w535 -> [w548 w580 w612]
                    tunnel: w534 -> [w547 w579 w611]
                    tunnel: w533 -> [w543 w575 w607]
                    tunnel: [w549 w581 w613] -> w532
                    tunnel: [w554 w586 w618] -> w531
                    tunnel: [w553 w585 w617] -> w530
                    tunnel: w528 -> [_ _ _]
                    tunnel: w527 -> [_ _ _]
                    tunnel: w526 -> [w538 w570 w602]
                    tunnel: w525 -> [w537 w569 w601]
                    tunnel: w524 -> [w536 w568 w600]
                    frame "I", "J", "U", "V", Default {
                      n140 = call "MLLF_WriteToBufferWithDelay.vi"("Delay Time ( 0,05 s)"=0.1 ("Command Time (s)"), "Command"="G0B1" ("String"), "Error In"=w547, "DriverConnect in"=w548) -> ("Error Out"=w544:errorcluster, "DriverConnect out"=w545:T1)  [unwired: 6 in]
                      n141 = for {
                        N: w543 -> [_]
                        tunnel: w545 -> [w564]
                        tunnel: w544 -> [w559]
                        tunnel: [w557] -> w541
                        tunnel: [w563] -> w550
                        tunnel: [w560] -> w549 mode=indexing
                        tunnel: w536 -> [w555]
                        stop <- w557 stop-if-true
                        n142 = case shown="\"H1\", Default" w555 {
                          tunnel: [1.5 ("Command Time (s)") 1.0 ("Command Time (s)") 2.0 ("Command Time (s)")] -> w556
                          frame "H1", Default {
                          }
                          frame "H0" {
                          }
                          frame "H2" {
                          }
                        }
                        n143 = call "Time Delay"("error in (no error)"=w559, "Delay Time (s)"=w556) -> ("error out"=w558:errorcluster)  [unwired: 9 in]
                        n144 = call "MLLF_ReadBuffer.vi"("Error In"=w558, "DriverConnect in"=w564) -> ("Error Out"=w557:errorcluster, "DriverConnect out"=w563:T1, "String"=w561:string)  [unwired: 6 in]
                        n145 = Fract/Exp String To Number(use system decimal point (T)=FALSE, string=w561) -> (number=w560:dbl)  [unwired: 2 in, 1 out]
                      }
                      n146 = call "Time Delay2"("error in (no error)"=w541, "Delay Time (s)"=0.1 ("Command Time (s)")) -> ("error out"=w540:errorcluster)  [unwired: 9 in]
                      n147 = call "B7_65_WriteAndCheck.vi"("DriverConnect in"=w550, "Str2Write"="G1B0" ("String"), "Command Time (s)"=0.1, "error in"=w540, "Driver Name"=w538, "Error Code"=w537) -> ("DriverConnect out"=w554:T1, "error out"=w553:T13)  [unwired: 8 in]
                    }
                    frame "F", "T" {
                      n148 = call "MLLF_WriteToBufferWithDelay.vi"("Delay Time ( 0,05 s)"=0.1 ("Command Time (s)"), "Command"="G0B1" ("String"), "Error In"=w579, "DriverConnect in"=w580) -> ("Error Out"=w576:errorcluster, "DriverConnect out"=w577:T1)  [unwired: 6 in]
                      n149 = for {
                        N: w575 -> [_]
                        tunnel: w577 -> [w596]
                        tunnel: w576 -> [w591]
                        tunnel: [w588] -> w573
                        tunnel: [w595] -> w582
                        tunnel: [w592] -> w581 mode=indexing
                        tunnel: w568 -> [w587]
                        stop <- w588 stop-if-true
                        n150 = case shown="\"H2\"" w587 {
                          tunnel: [1.0 ("Command Time (s)") 1.0 ("Command Time (s)") 1.0 ("Command Time (s)")] -> w589
                          frame "H1", Default {
                          }
                          frame "H0" {
                          }
                          frame "H2" {
                          }
                        }
                        n151 = call "Time Delay5"("error in (no error)"=w591, "Delay Time (s)"=w589) -> ("error out"=w590:errorcluster)  [unwired: 9 in]
                        n152 = call "MLLF_ReadBuffer.vi"("Error In"=w590, "DriverConnect in"=w596) -> ("Error Out"=w588:errorcluster, "DriverConnect out"=w595:T1, "String"=w593:string)  [unwired: 6 in]
                        n153 = Fract/Exp String To Number(use system decimal point (T)=FALSE, string=w593) -> (number=w592:dbl)  [unwired: 2 in, 1 out]
                      }
                      n154 = call "Time Delay6"("error in (no error)"=w573, "Delay Time (s)"=0.1 ("Command Time (s)")) -> ("error out"=w572:errorcluster)  [unwired: 9 in]
                      n155 = call "B7_65_WriteAndCheck.vi"("DriverConnect in"=w582, "Str2Write"="G1B0" ("String"), "Command Time (s)"=0.1, "error in"=w572, "Driver Name"=w570, "Error Code"=w569) -> ("DriverConnect out"=w586:T1, "error out"=w585:T13)  [unwired: 8 in]
                    }
                    frame "R", "Z" {
                      n156 = call "MLLF_WriteToBufferWithDelay.vi"("Delay Time ( 0,05 s)"=0.1 ("Command Time (s)"), "Command"="G0B1" ("String"), "Error In"=w611, "DriverConnect in"=w612) -> ("Error Out"=w608:errorcluster, "DriverConnect out"=w609:T1)  [unwired: 6 in]
                      n157 = for {
                        N: w607 -> [_]
                        tunnel: w609 -> [w628]
                        tunnel: w608 -> [w623]
                        tunnel: [w621] -> w605
                        tunnel: [w627] -> w614
                        tunnel: [w624] -> w613 mode=indexing
                        tunnel: w600 -> [w620]
                        stop <- w621 stop-if-true
                        n158 = case shown="\"H1\", Default" w620 {
                          tunnel: [2.5 ("Command Time (s)") 2.0 ("Command Time (s)") 4.0 ("Command Time (s)")] -> w619
                          frame "H1", Default {
                          }
                          frame "H0" {
                          }
                          frame "H2" {
                          }
                        }
                        n159 = call "Time Delay3"("error in (no error)"=w623, "Delay Time (s)"=w619) -> ("error out"=w622:errorcluster)  [unwired: 9 in]
                        n160 = call "MLLF_ReadBuffer.vi"("Error In"=w622, "DriverConnect in"=w628) -> ("Error Out"=w621:errorcluster, "DriverConnect out"=w627:T1, "String"=w625:string)  [unwired: 6 in]
                        n161 = Fract/Exp String To Number(use system decimal point (T)=FALSE, string=w625) -> (number=w624:dbl)  [unwired: 2 in, 1 out]
                      }
                      n162 = call "Time Delay4"("error in (no error)"=w605, "Delay Time (s)"=0.1 ("Command Time (s)")) -> ("error out"=w604:errorcluster)  [unwired: 9 in]
                      n163 = call "B7_65_WriteAndCheck.vi"("DriverConnect in"=w614, "Str2Write"="G1B0" ("String"), "Command Time (s)"=0.1, "error in"=w604, "Driver Name"=w602, "Error Code"=w601) -> ("DriverConnect out"=w618:T1, "error out"=w617:T13)  [unwired: 8 in]
                    }
                  }
                }
              }
              n164 = call "MLLF_ClearBuffer.vi"("Timeout(default = 300 ms)"=u32 300 ("Timeout"), "Error In"=w449, "DriverConnect in"=w450) -> ("Error Out"=w459:errorcluster)  [unwired: 5 in, 2 out]
              n165 = Delete From Array(array=w451, length=0, index=0) -> (array with subset deleted=w446:dbl[])  [unwired: 1 out]
            }
          }
          n166 = call "MLLF_FormatOutputValueWithUnits.vi"("Format"="%.;%^#_7e" ("format string"), "error in"=w418, "ValuesIn"=w424) -> ("error out"=w416:T13, "Result string"=w417:T14)  [unwired: 7 in]
        }
        frame "close" {
          n167 = Unbundle By Name(w633) -> ("Data.Connect.OpenedSession"=w635:T3)
          n168 = VISA Close(VISA resource name=w635) -> (error out=w634:errorcluster)  [unwired: 1 in]
        }
      }
    }
    frame Error {
    }
  }
  n169 = local write "Settings"(w9) -> ()
  n170 = flat-sequence {
    tunnel: [w646] -> w3
    tunnel: [w645] -> w1
    tunnel: w6 -> [w644]
    tunnel: w4 -> [w643]
    tunnel: w5 -> [w639]
    tunnel: [w641] -> w2
    frame #0 {
      # "driver out"
      n171 = Unbundle By Name(w639) -> ("Data"=w638:T15)
      n172 = To Variant(anything=w638) -> (Variant=w640:variant)
      n173 = Bundle By Name(cluster=w639, "Saved Data"=w640) -> (w641:T7)
      n174 = call "MLLF_SaveLastSettingUtility.vi"("error in"=w643, "Saved Data"=w640) -> ("error out"=w642:T13)  [unwired: 8 in, 1 out]
      n175 = call "MCF_Output.vi"("Error In"=w642, "Input"=w644) -> ("Error Out"=w645:errorcluster, "Output"=w646:string)  [unwired: 8 in]
    }
  }
  n176 = local write "Settings"(w2) -> ()
  "error out" <- w1
  "Response" <- w3
